vi "test Add Import Deploy.vi"(8 "error in":errorcluster, 11 "TestCase in":refnum<class "Examples.lvclass">) -> (0 "error out":errorcluster, 3 "TestCase out":refnum<class "Examples.lvclass">)   [LabVIEW 2020, in "Examples.lvclass"]
uses:
  Examples.lvclass
  Examples.lvclass/Examples.ctl
  <vilib>/addons/_JKI Toolkits/VI Tester/TestCase.llb/TestCase.lvclass
  7f6914e5-79d7-41a5-a6cd-be6651e4326d.vi
  C:/Program Files (x86)/National Instruments/LabVIEW 2020/vi.lib/addons/_JKI Toolkits/VI Tester/TestCase.llb/TestCase.lvclass
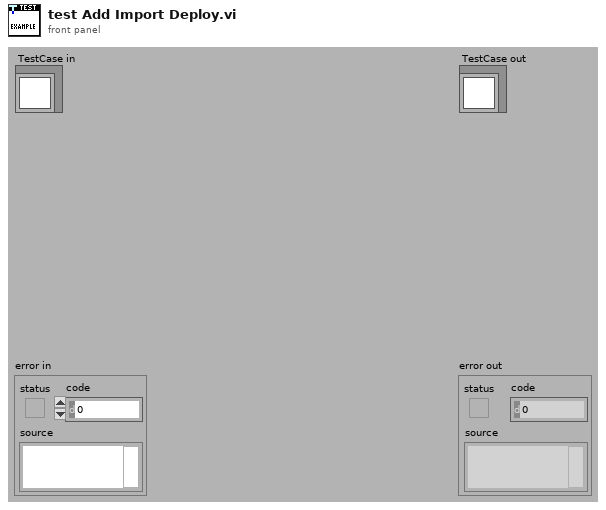
[diagram p1: front panel]
types:
  T1 = typedef "NI_VS Workspace ExecutionAPI.lvlib/WorkspaceAPI.ctl" = refnum<k24>
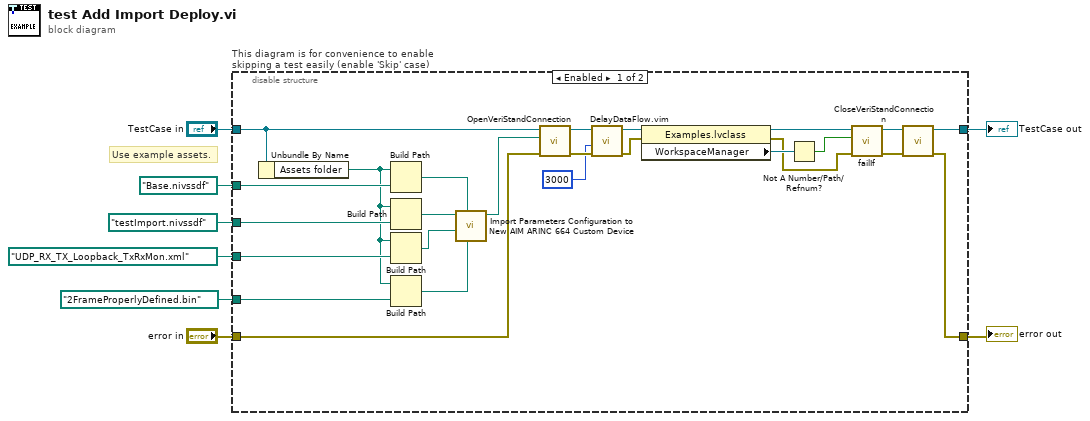
[diagram p0: block diagram]
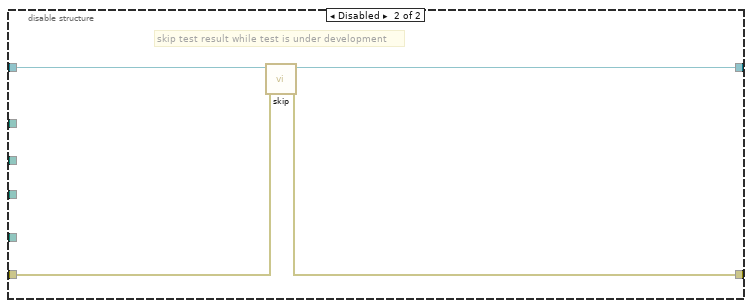
[diagram p2: hidden frame]
diagram:
  # "Use example assets."
  n1 = disable-structure "This diagram is for convenience to enable skipping a test easily (enable 'Skip' case)" shown="Enabled" {
    disable-tunnel: "TestCase in" -> [w19 w36]
    disable-tunnel: [w20 w34] -> w5
    disable-tunnel: [w21 w35] -> w7
    disable-tunnel: "error in" -> [w18 w33]
    disable-tunnel: path "UDP_RX_TX_Loopback_TxRxMon.xml" ("name or relative path") -> [w32 _]
    disable-tunnel: path "Base.nivssdf" ("name or relative path") -> [w16 _]
    disable-tunnel: path "testImport.nivssdf" ("name or relative path") -> [w15 _]
    disable-tunnel: path "2FrameProperlyDefined.bin" ("name or relative path") -> [w9 _]
    frame Enabled {
      n2 = Unbundle By Name(w19) -> ("Assets folder"=w11:path)
      n3 = Build Path(base path=w11, name or relative path=w16) -> (appended path=w13:path)
      n4 = Build Path(base path=w11, name or relative path=w15) -> (appended path=w14:path)
      n5 = Build Path(base path=w11, name or relative path=w32) -> (appended path=w12:path)
      n6 = Build Path(base path=w11, name or relative path=w9) -> (appended path=w10:path)
      n7 = call "Import Parameters Configuration to New AIM ARINC 664 Custom Device.vi"("Bin File Parameter Data"=w10, "Base System Definition File"=w13, "Parameters Configuration File"=w12, "Output System Definition File"=w14) -> ("AIM ARINC 664 System Definition"=w17:path)  [unwired: 7 in]
      n8 = call-dynamic "OpenVeriStandConnection.vi"("error in (no error)"=w18, "System Definition File"=w17, "VeriStand Test Case in"=w19) -> ("error out"=w24:errorcluster, "VeriStand Test Case out"=w23:refnum<class "Examples.lvclass">)  [unwired: 6 in, 1 out]
      n9 = call "DelayDataFlow.vim"("value in"=w24, "milliseconds to wait"=u32 3000) -> ("value out"=w31:errorcluster)  [unwired: 2 in, 1 out]
      n10 = property class="Examples.lvclass"(reference=w23, error in=w31) -> (reference out=w30:refnum<class "Examples.lvclass">, error out=w25:errorcluster, "WorkspaceManager"=w27:T1)
      n11 = Not A Number/Path/Refnum?(number/path/refnum=w27) -> (NaN/Path/Refnum?=w26:bool)
      n12 = call-dynamic "failIf.vi"("error in (no error)"=w25, "fail"=w26, "TestCase in"=w30) -> ("error out"=w28:errorcluster, "TestCase out"=w29:refnum<class "Examples.lvclass">)  [unwired: 7 in]
      n13 = call-dynamic "CloseVeriStandConnection.vi"("error in (no error)"=w28, "VeriStand Test Case in"=w29) -> ("error out"=w21:errorcluster, "VeriStand Test Case out"=w20:refnum<class "Examples.lvclass">)  [unwired: 8 in]
    }
    frame Disabled {
      # "skip test result while test is under development"
      n14 = call <vilib>:"skip.vi"("error in (no error)"=w33, "TestCase in"=w36) -> ("error out"=w35:errorcluster, "TestCase out"=w34:refnum<class "Examples.lvclass">)  [unwired: 8 in]
    }
  }
  "error out" <- w7
  "TestCase out" <- w5
